vi "RemapIcon.vi"() -> ()   [LabVIEW 2014]
uses:
  <vilib>/picture/picture.llb/imagedata.ctl
panel:
  out "image 2":u8[](array[numeric])
  out "output cluster":T1
  in  "image":u8[](array[numeric])=[0, 0, 0, 0, 255, 255, 255, 255, 255, 255, 255, 255, 255, 255, 255, 255, 0, 0, 0, 255, 0, 0, 0, 255, 1, 1, 1, 1, 1, 1, 1, 255, 255, 1, 255, 255, 0, 0, 0, 255, 0, 0, 255, 1, 255, 255, 1, 255, 255, 1, 1, 255, 1, 255, 1, 255, 0, 0, 0, 0, 0, 255, 1, 255, 1, 1, 1, 1, 1, 1, 1, 1, 255, 1, 1, 255, 0, 0, 0, 23, 255, 255, 255, 255, 255, 255, 255, 255, 255, 255, 255, 255, 1, 1, 1, 255, 0, 0, 0, 23, 255, 1, 1, 1, 1, 1, 1, 1, 1, 1, 1, 255, 1, 1, 1, 255, 0, 0, 0, 0, 255, 1, 1, 1, 1, 1, 1, 1, 255, 255, 255, 255, 255, 255, 255, 255, 255, 255, 255, 255, 255, 1, 1, 255, 255, 1, 1, 255, 1, 1, 1, 1, 1, 1, 255, 255, 1, 255, 255, 255, 255, 1, 1, 255, 255, 1, 255, 1, 255, 255, 1, 255, 255, 1, 255, 1, 255, 1, 255, 255, 255, 1, 1, 1, 1, 255, 1, 255, 1, 1, 1, 1, 1, 1, 1, 255, 1, 1, 255, 0, 255, 1, 1, 1, 255, 255, 255, 255, 255, 255, 255, 255, 255, 255, 255, 1, 1, 1, 255, 23, 255, 1, 1, 1, 255, 1, 1, 1, 1, 1, 1, 1, 1, 1, 255, 1, 1, 1, 255, 23, 255, 1, 1, 1, 255, 1, 1, 1, 1, 1, 1, 1, 1, 1, 255, 1, 255, 1, 255, 0, 255, 1, 1, 1, 255, 1, 1, 1, 1, 1, 255, 255, 1, 1, 255, 1, 255, 1, 255, 255, 255, 1, 1, 1, 255, 1, 1, 1, 1, 1, 255, 255, 1, 1, 255, 1, 1, 1, 255, 255, 255, 255, 255, 255, 255, 1, 1, 1, 1, 1, 1, 1, 1, 1, 255, 1, 1, 1, 255, 255, 0, 0, 0, 0, 255, 1, 1, 255, 255, 1, 1, 1, 1, 1, 255, 1, 1, 1, 255, 0, 0, 0, 0, 0, 255, 1, 1, 255, 255, 1, 1, 1, 1, 1, 255, 1, 1, 255, 0, 23, 0, 0, 0, 0, 255, 1, 1, 1, 1, 1, 1, 1, 1, 1, 255, 1, 255, 0, 0, 23, 0, 0, 0, 0, 255, 1, 1, 1, 1, 1, 1, 1, 1, 1, 255, 255, 0, 0, 0, 0, 0, 0, 0, 0, 255, 255, 255, 255, 255, 255, 255, 255, 255, 255, 255, 0, 0, 0, 0, 255]
  out "new picture 2":picture
  out "new picture":picture
  out "Array 2":i32[](array[numeric])
  out "Array 5":i32[](array[numeric])
  in  "Image Data":T1={"image type"=0, "image depth"=8, "image"=[0, 0, 0, 0, 255, 255, 255, 255, 255, 255, 255, 255, 255, 255, 255, 255, 0, 0, 0, 255, 0, 0, 0, 255, 1, 1, 1, 1, 1, 1, 1, 255, 255, 1, 255, 255, 0, 0, 0, 255, 0, 0, 255, 1, 255, 255, 1, 255, 255, 1, 1, 255, 1, 255, 1, 255, 0, 0, 0, 0, 0, 255, 1, 255, 1, 1, 1, 1, 1, 1, 1, 1, 255, 1, 1, 255, 0, 0, 0, 23, 255, 255, 255, 255, 255, 255, 255, 255, 255, 255, 255, 255, 1, 1, 1, 255, 0, 0, 0, 23, 255, 1, 1, 1, 1, 1, 1, 1, 1, 1, 1, 255, 1, 1, 1, 255, 0, 0, 0, 0, 255, 1, 1, 1, 1, 1, 1, 1, 255, 255, 255, 255, 255, 255, 255, 255, 255, 255, 255, 255, 255, 1, 1, 255, 255, 1, 1, 255, 1, 1, 1, 1, 1, 1, 255, 255, 1, 255, 255, 255, 255, 1, 1, 255, 255, 1, 255, 1, 255, 255, 1, 255, 255, 1, 255, 1, 255, 1, 255, 255, 255, 1, 1, 1, 1, 255, 1, 255, 1, 1, 1, 1, 1, 1, 1, 255, 1, 1, 255, 0, 255, 1, 1, 1, 255, 255, 255, 255, 255, 255, 255, 255, 255, 255, 255, 1, 1, 1, 255, 23, 255, 1, 1, 1, 255, 1, 1, 1, 1, 1, 1, 1, 1, 1, 255, 1, 1, 1, 255, 23, 255, 1, 1, 1, 255, 1, 1, 1, 1, 1, 1, 1, 1, 1, 255, 1, 255, 1, 255, 0, 255, 1, 1, 1, 255, 1, 1, 1, 1, 1, 255, 255, 1, 1, 255, 1, 255, 1, 255, 255, 255, 1, 1, 1, 255, 1, 1, 1, 1, 1, 255, 255, 1, 1, 255, 1, 1, 1, 255, 255, 255, 255, 255, 255, 255, 1, 1, 1, 1, 1, 1, 1, 1, 1, 255, 1, 1, 1, 255, 255, 0, 0, 0, 0, 255, 1, 1, 255, 255, 1, 1, 1, 1, 1, 255, 1, 1, 1, 255, 0, 0, 0, 0, 0, 255, 1, 1, 255, 255, 1, 1, 1, 1, 1, 255, 1, 1, 255, 0, 23, 0, 0, 0, 0, 255, 1, 1, 1, 1, 1, 1, 1, 1, 1, 255, 1, 255, 0, 0, 23, 0, 0, 0, 0, 255, 1, 1, 1, 1, 1, 1, 1, 1, 1, 255, 255, 0, 0, 0, 0, 0, 0, 0, 0, 255, 255, 255, 255, 255, 255, 255, 255, 255, 255, 255, 0, 0, 0, 0, 255], "mask"=[], "colors"=[16777215, 16777164, 16777113, 16777062, 16777011, 16776960, 16764159, 16764108, 16764057, 16764006, 16763955, 16763904, 16751103, 16751052, 16751001, 16750950, 16750899, 16750848, 16738047, 16737996, 16737945, 16737894, 16737843, 16737792, 16724991, 16724940, 16724889, 16724838, 16724787, 16724736, 16711935, 16711884, 16711833, 16711782, 16711731, 16711680, 13434879, 13434828, 13434777, 13434726, 13434675, 13434624, 13421823, 13421772, 13421721, 13421670, 13421619, 13421568, 13408767, 13408716, 13408665, 13408614, 13408563, 13408512, 13395711, 13395660, 13395609, 13395558, 13395507, 13395456, 13382655, 13382604, 13382553, 13382502, 13382451, 13382400, 13369599, 13369548, 13369497, 13369446, 13369395, 13369344, 10092543, 10092492, 10092441, 10092390, 10092339, 10092288, 10079487, 10079436, 10079385, 10079334, 10079283, 10079232, 10066431, 10066380, 10066329, 10066278, 10066227, 10066176, 10053375, 10053324, 10053273, 10053222, 10053171, 10053120, 10040319, 10040268, 10040217, 10040166, 10040115, 10040064, 10027263, 10027212, 10027161, 10027110, 10027059, 10027008, 6750207, 6750156, 6750105, 6750054, 6750003, 6749952, 6737151, 6737100, 6737049, 6736998, 6736947, 6736896, 6724095, 6724044, 6723993, 6723942, 6723891, 6723840, 6711039, 6710988, 6710937, 6710886, 6710835, 6710784, 6697983, 6697932, 6697881, 6697830, 6697779, 6697728, 6684927, 6684876, 6684825, 6684774, 6684723, 6684672, 3407871, 3407820, 3407769, 3407718, 3407667, 3407616, 3394815, 3394764, 3394713, 3394662, 3394611, 3394560, 3381759, 3381708, 3381657, 3381606, 3381555, 3381504, 3368703, 3368652, 3368601, 3368550, 3368499, 3368448, 3355647, 3355596, 3355545, 3355494, 3355443, 3355392, 3342591, 3342540, 3342489, 3342438, 3342387, 3342336, 65535, 65484, 65433, 65382, 65331, 65280, 52479, 52428, 52377, 52326, 52275, 52224, 39423, 39372, 39321, 39270, 39219, 39168, 26367, 26316, 26265, 26214, 26163, 26112, 13311, 13260, 13209, 13158, 13107, 13056, 255, 204, 153, 102, 51, 15597568, 14483456, 12255232, 11141120, 8912896, 7798784, 5570560, 4456448, 2228224, 1114112, 60928, 56576, 47872, 43520, 34816, 30464, 21760, 17408, 8704, 4352, 238, 221, 187, 170, 136, 119, 85, 68, 34, 17, 15658734, 14540253, 12303291, 11184810, 8947848, 7829367, 5592405, 4473924, 2236962, 1118481, 0], "Rectangle"={"left"=0, "top"=0, "right"=19, "bottom"=21}}
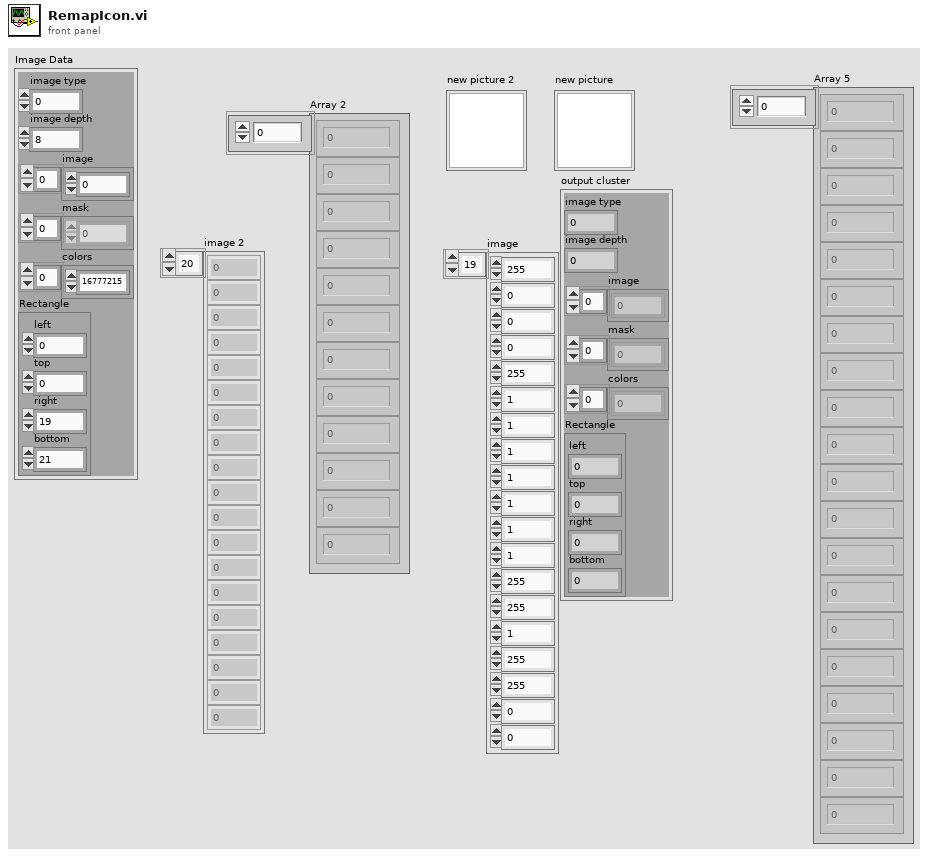
[diagram p1: front panel]
types:
  T1 = typedef "imagedata.ctl" = cluster{"image type":i32, "image depth":i32, "image":u8[], "mask":u8[], "colors":u32[], "Rectangle":cluster{"left":i16, "top":i16, "right":i16, "bottom":i16}}
  T2 = cluster{"left":i16, "top":i16, "right":i16, "bottom":i16}
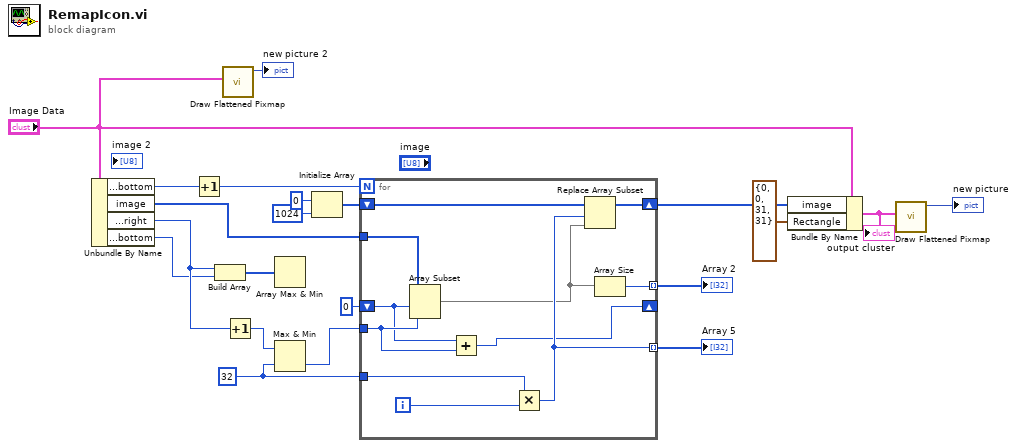
[diagram p0: block diagram]
diagram:
  w3 = i16 32 ("Rectangle.right")
  n1 = Unbundle By Name("Image Data") -> ("Rectangle.bottom"=w6:i16, "image"=w18:u8[], "Rectangle.right"=w7:i16, "Rectangle.bottom"=w5:i16)
  n2 = Increment(x=w6) -> (x+1=w4:i16)
  n3 = Build Array(w7, w5) -> (w11:i16[])
  n4 = call <vilib>:"Draw Flattened Pixmap.vi"("image data"="Image Data") -> ("new picture"=→"new picture 2":picture)  [unwired: 8 in]
  n5 = Increment(x=w7) -> (x+1=w2:i16)
  n6 = Array Max & Min(array=w11) -> ()  [unwired: 4 out]
  n7 = Max & Min(x=w2, y=w3) -> (min(x,y)=w1:i16)  [unwired: 1 out]
  n8 = Initialize Array(u8 0, 1024 ("dimension size")) -> (w19:u8[])
  n9 = for {
    N: w4 -> [_]
    tunnel: w18 -> [w27]
    shift-right: [w31] -> w17
    shift-left: w19 -> [w32]
    tunnel: w3 -> [w30]
    shift-right: [w23] -> _
    shift-left: 0 -> [w24]
    tunnel: w1 -> [w25]
    tunnel: [w29] -> w13 mode=indexing
    tunnel: [w28] -> w12 mode=indexing
    i -> [w26]
    n10 = Array Subset(array=w27, index=w24, length=w25) -> (w22:u8[])
    n11 = Add(x=w24, y=w25) -> (x+y=w23:i32)
    n12 = Multiply(x=w30, y=w26) -> (x*y=w28:i32)
    n13 = Replace Array Subset(array=w32, new element=w22, index=w28) -> (w31:u8[])
    n14 = Array Size(array=w22) -> (size(s)=w29:i32)
  }
  "Array 2" <- w13
  "Array 5" <- w12
  n15 = Bundle By Name(cluster="Image Data", "image"=w17, "Rectangle"=T2 {"left"=0, "top"=0, "right"=31, "bottom"=31}) -> (w16:T1)
  "output cluster" <- w16
  n16 = call <vilib>:"Draw Flattened Pixmap.vi"("image data"=w16) -> ("new picture"=→"new picture":picture)  [unwired: 8 in]
